vi "FlexDDS-NG_DCP_WriteCFR1_C.vi"(6 "Internal profile control":T1(ring), 8 "RAM playback destination":T2(ring), 9 "CFR1 bits":T3={"RAM enable (F)"=FALSE, "Manual OSK external control (F)"=FALSE, "Inverse sinc filter enable (T)"=TRUE, "DDS sine (/cosine) output (F)"=FALSE, "Load LRR at I/O update (F)"=FALSE, "Autoclear digital ramp accumulator (F)"=FALSE, "Autoclear phase accumulator (F)"=FALSE, "Clear digital ramp accumulator (F)"=FALSE, "Clear phase accumulator (F)"=FALSE, "Load ARR at I/O update (F)"=FALSE, "OSK enable (F)"=FALSE, "Select Auto OSK (F)"=FALSE}, 10 "Channels":T4(ring)=enum."Both channels", 11 "initial instruction string":string) -> (3 "appended instruction string":string="dcp spi:CFR1=0x400000\r")   [LabVIEW 2010]
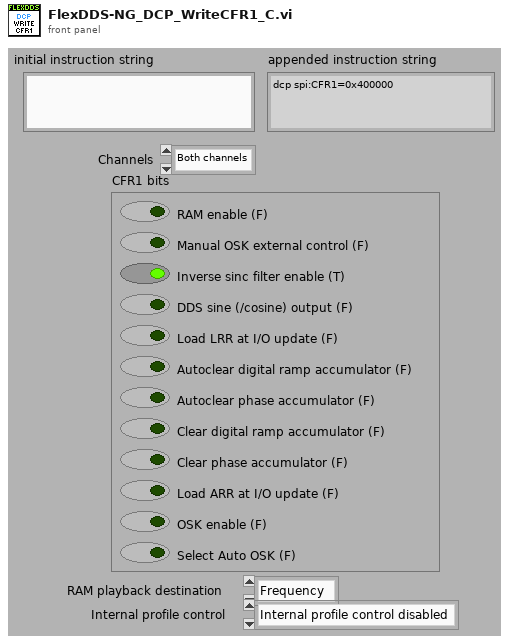
[diagram p1: front panel]
types:
  T1 = enum32{"Internal profile control disabled", "Execute profile 0 to 1, then halt", "Execute profile 0 to 2, then halt", "Execute profile 0 to 3, then halt", "Execute profile 0 to 4, then halt", "Execute profile 0 to 5, then halt", "Execute profile 0 to 6, then halt", "Execute profile 0 to 7, then halt", "Execute profile 0 to 1, continuously", "Execute profile 0 to 2, continuously", "Execute profile 0 to 3, continuously", "Execute profile 0 to 4, continuously", "Execute profile 0 to 5, continuously", "Execute profile 0 to 6, continuously", "Execute profile 0 to 7, continuously", ""}
  T2 = enum32{"Frequency", "Phase", "Amplitude", "Polar"}
  T3 = cluster{"RAM enable (F)":bool, "Manual OSK external control (F)":bool, "Inverse sinc filter enable (T)":bool, "DDS sine (/cosine) output (F)":bool, "Load LRR at I/O update (F)":bool, "Autoclear digital ramp accumulator (F)":bool, "Autoclear phase accumulator (F)":bool, "Clear digital ramp accumulator (F)":bool, "Clear phase accumulator (F)":bool, "Load ARR at I/O update (F)":bool, "OSK enable (F)":bool, "Select Auto OSK (F)":bool}
  T4 = enum32{"Channel 0", "Channel 1", "Both channels"}
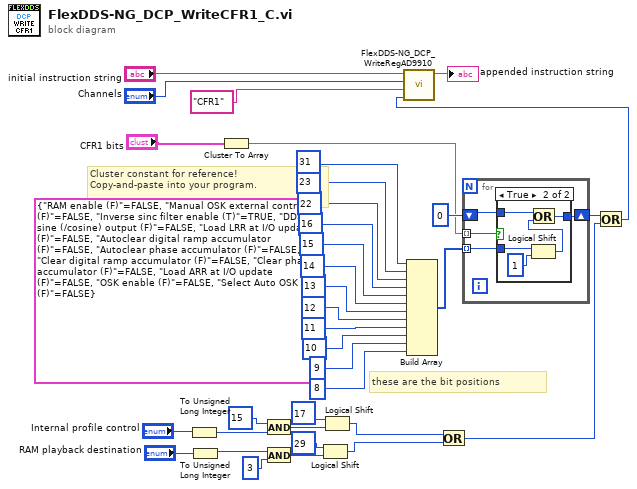
[diagram p0: block diagram]
diagram:
  (unwired) T3 {"RAM enable (F)"=FALSE, "Manual OSK external control (F)"=FALSE, "Inverse sinc filter enable (T)"=TRUE, "DDS sine (/cosine) output (F)"=FALSE, "Load LRR at I/O update (F)"=FALSE, "Autoclear digital ramp accumulator (F)"=FALSE, "Autoclear phase accumulator (F)"=FALSE, "Clear digital ramp accumulator (F)"=FALSE, "Clear phase accumulator (F)"=FALSE, "Load ARR at I/O update (F)"=FALSE, "OSK enable (F)"=FALSE, "Select Auto OSK (F)"=FALSE} ("Cluster")
  # "these are the bit positions"
  # "Cluster constant for reference!\nCopy-and-paste into your program."
  n1 = To Unsigned Long Integer(number="Internal profile control") -> (unsigned 32bit integer=w1:u32)
  n2 = To Unsigned Long Integer(number="RAM playback destination") -> (unsigned 32bit integer=w13:u32)
  n3 = Cluster To Array(cluster="CFR1 bits") -> (array=w16:bool[])
  n4 = And(x=u32 15, y=w1) -> (x .and. y?=w8:u32)
  n5 = And(x=w13, y=u32 3) -> (x .and. y?=w11:u32)
  n6 = Logical Shift(y=i8 29, x=w11) -> (x << y=w9:u32)
  n7 = Logical Shift(y=i8 17, x=w8) -> (x << y=w6:u32)
  n8 = Build Array(31 ("single tone profile (0..7)"), 23 ("single tone profile (0..7)"), 22 ("single tone profile (0..7)"), 16 ("single tone profile (0..7)"), 15 ("single tone profile (0..7)"), 14 ("single tone profile (0..7)"), 13 ("single tone profile (0..7)"), 12 ("single tone profile (0..7)"), 11 ("single tone profile (0..7)"), 10 ("single tone profile (0..7)"), 9 ("single tone profile (0..7)"), 8 ("single tone profile (0..7)")) -> (w19:i32[])
  n9 = Or(x=w6, y=w9) -> (x .or. y?=w4:u32)
  n10 = for {
    tunnel: w16 -> [w36] mode=indexing
    tunnel: w19 -> [w39] mode=indexing
    shift-right: [w38] -> w5
    shift-left: u32 0 ("x") -> [w37]
    n11 = case shown="True" w36 {
      tunnel: w39 -> [_ w45]
      tunnel: [w40 w42] -> w38
      tunnel: w37 -> [w40 w41]
      frame False {
      }
      frame True {
        n12 = Logical Shift(y=w45, x=u32 1) -> (x << y=w43:u32)
        n13 = Or(x=w41, y=w43) -> (x .or. y?=w42:u32)
      }
    }
  }
  n14 = Or(x=w5, y=w4) -> (x .or. y?=w3:u32)
  n15 = call "FlexDDS-NG_DCP_WriteRegAD9910.vi"("register content"=w3, "AD9910 register name"="CFR1" ("format string"), "Channels"="Channels", "initial instruction string"="initial instruction string") -> ("appended instruction string"=→"appended instruction string":string)  [unwired: 7 in]
